vi "command_receiver.vi"() -> ()   [LabVIEW 2023]
uses:
  Command Generic.ctl
panel:
  out "ACK sent":string
  out "RAW Data":string
  out "remote address":string
  out "Data 11":string
  out "Data 9":string
  out "Data 12":string
  out "Data 10":string
  out "Data 8":string
  out "Data 7":string
  out "Data 6":string
  out "Data 5":string
  out "Data 4":string
  out "Data 3":string
  out "Data 2":string
  out "Data 1":string
  in  "Abort":bool
  in  "PORT":u16=7704
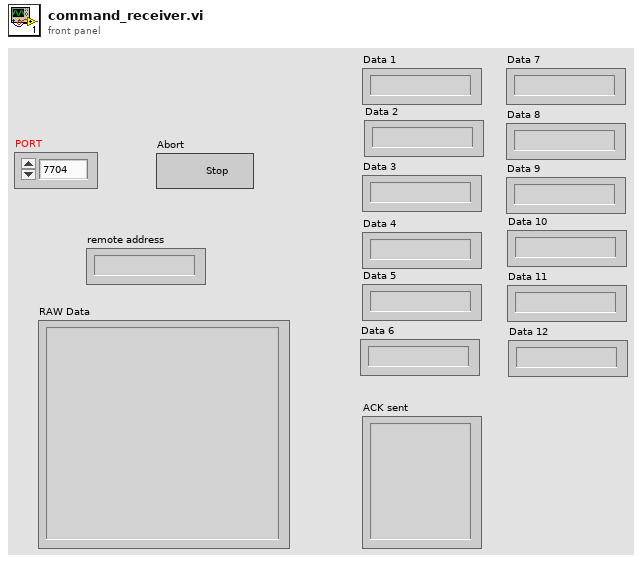
[diagram p1: front panel]
types:
  T1 = typedef "Command Generic.ctl" = cluster{"Data 1":string, "Data 2":string, "Data 3":string, "Data 4":string, "Data 5":string, "Data 6":string, "Data 7":string, "Data 8":string, "Data 9":string, "Data 10":string, "Data 11":string, "Data 12":string}
  T2 = enum16{"Standard", "Buffered", "CRLF", "Immediate"}
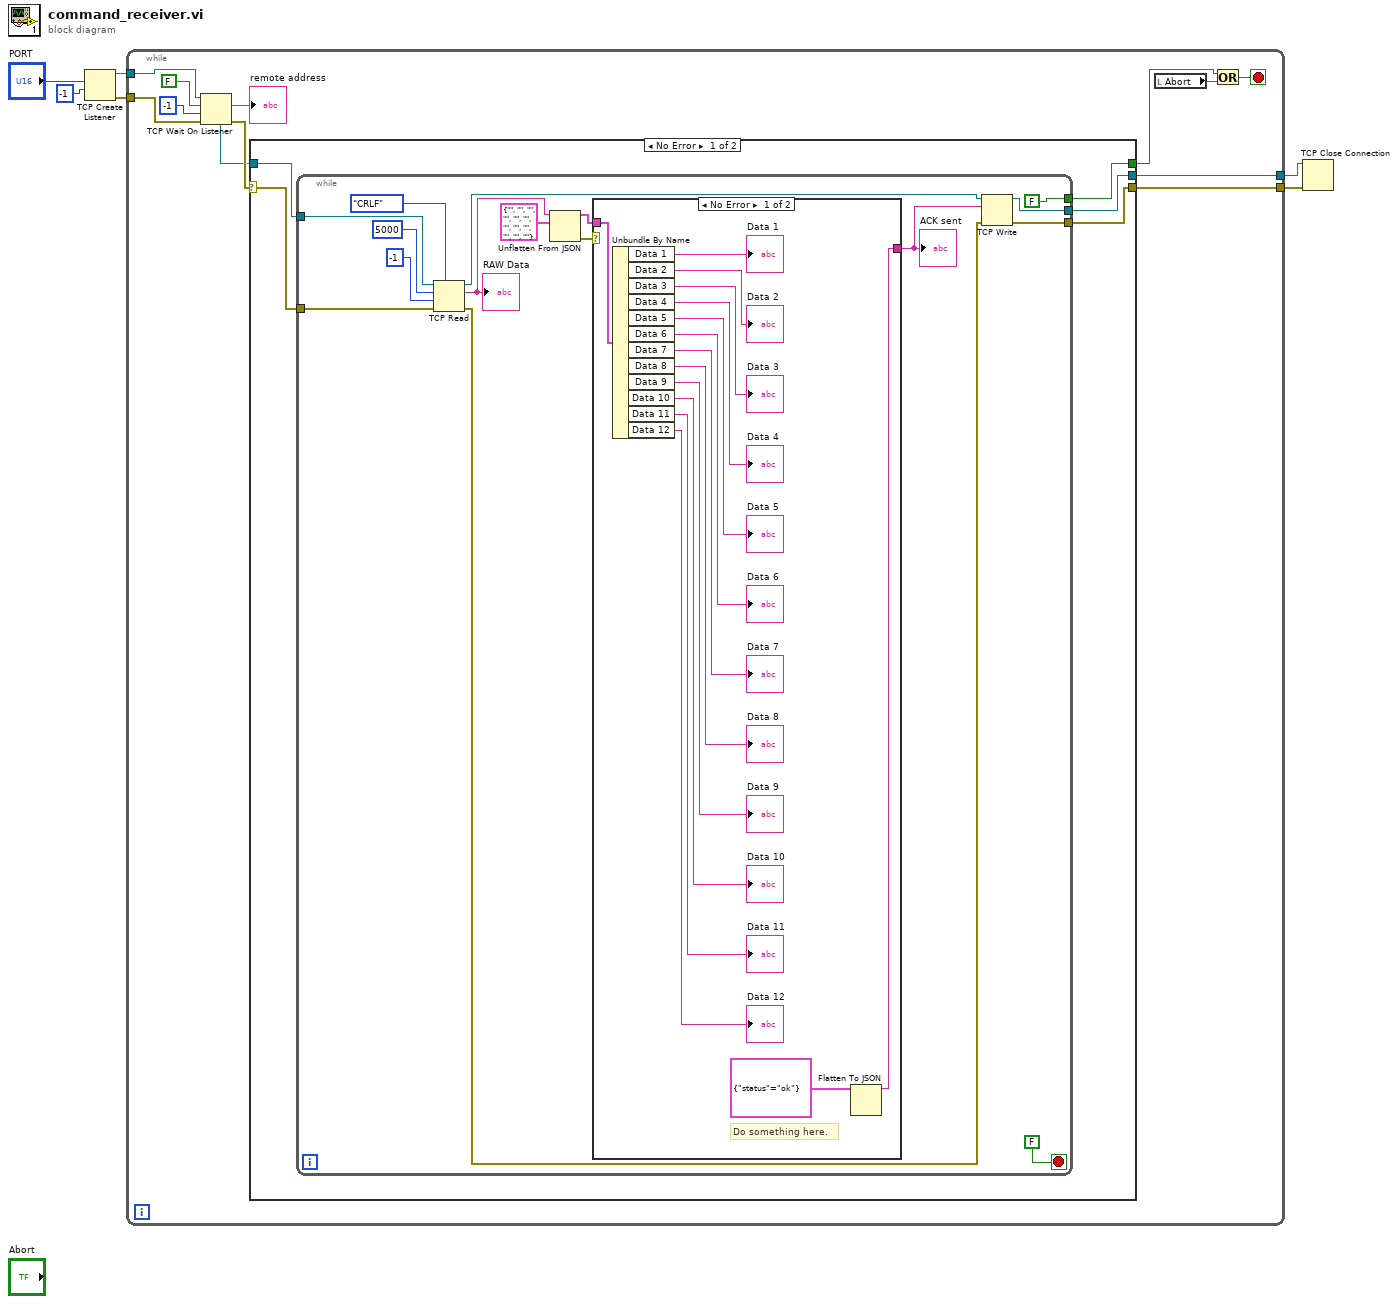
[diagram p0: block diagram]
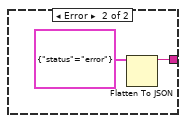
[diagram p2: hidden frame]
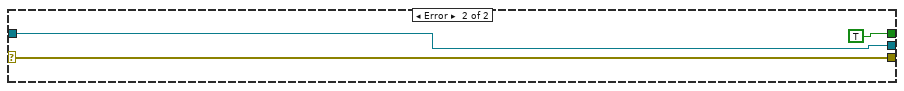
[diagram p3: hidden frame]
diagram:
  n1 = TCP Create Listener(9:-1 ("timeout ms (25000)"), 10:"PORT") -> (0:w3:errorcluster, 3:w4:refnum<k5>)  [unwired: 3 in, 1 out]
  n2 = while {
    tunnel: w4 -> [w18]
    tunnel: w3 -> [w17]
    tunnel: [w15] -> w2
    tunnel: [w7] -> w1
    stop <- w13 stop-if-true
    n3 = TCP Wait On Listener(8:w17, 9:-1 ("timeout ms (wait forever: -1)"), 10:FALSE ("resolve remote address (T)"), 11:w18) -> (0:w16:errorcluster, 2:→"remote address":string, 4:w8:refnum<k5>)  [unwired: 2 out]
    n4 = case shown="No Error" w16 {
      selector: w16 -> [w23 w58]
      tunnel: [w22 w58] -> w15
      tunnel: [w21 TRUE] -> w14
      tunnel: w8 -> [w20 w57]
      tunnel: [w19 w57] -> w7
      frame No Error {
        n5 = while {
          tunnel: [FALSE] -> w21
          tunnel: [w34] -> w19
          tunnel: w23 -> [w38]
          tunnel: [w32] -> w22
          tunnel: w20 -> [w24]
          stop <- FALSE stop-if-true
          n6 = TCP Read(connection ID=w24, bytes to read=5000, error in (no error)=w38, 7:T2."CRLF" ("mode (standard)"), 9:-1 ("timeout ms (25000)")) -> (connection ID out=w30:refnum<k5>, data out=w28:string, error out=w33:errorcluster)
          "RAW Data" <- w28
          n7 = Unflatten From JSON(JSON string=w28, type and defaults=T1 {"Data 1"="", "Data 2"="", "Data 3"="", "Data 4"="", "Data 5"="", "Data 6"="", "Data 7"="", "Data 8"="", "Data 9"="", "Data 10"="", "Data 11"="", "Data 12"=""} ("Command Generic")) -> (value=w26:T1, error out=w35:errorcluster)  [unwired: 5 in]
          n8 = case shown="No Error" w35 {
            tunnel: [w53 w55] -> w25
            tunnel: w26 -> [w52 _]
            frame No Error {
              # "Do something here."
              n9 = Unbundle By Name(w52) -> ("Data 1"=→"Data 1":string, "Data 2"=→"Data 2":string, "Data 3"=→"Data 3":string, "Data 4"=→"Data 4":string, "Data 5"=→"Data 5":string, "Data 6"=→"Data 6":string, "Data 7"=→"Data 7":string, "Data 8"=→"Data 8":string, "Data 9"=→"Data 9":string, "Data 10"=→"Data 10":string, "Data 11"=→"Data 11":string, "Data 12"=→"Data 12":string)
              n10 = Flatten To JSON(anything=cluster{"status":string} {"status"="ok"}) -> (JSON string=w53:string)  [unwired: 2 in, 1 out]
            }
            frame Error {
              n11 = Flatten To JSON(anything=cluster{"status":string} {"status"="error"}) -> (JSON string=w55:string)  [unwired: 2 in, 1 out]
            }
          }
          "ACK sent" <- w25
          n12 = TCP Write(connection ID=w30, data in=w25, error in (no error)=w33) -> (connection ID out=w34:refnum<k5>, error out=w32:errorcluster)  [unwired: 1 in, 1 out]
        }
      }
      frame Error {
      }
    }
    n13 = local read "Abort"() -> (w12:bool)
    n14 = Or(x=w14, y=w12) -> (x .or. y?=w13:bool)
  }
  n15 = TCP Close Connection(connection ID=w1, error in (no error)=w2) -> ()  [unwired: 1 in, 2 out]
